vi "read file.vi"() -> ()   [LabVIEW 2011]
panel:
  out "Image":T1(plugin-control)
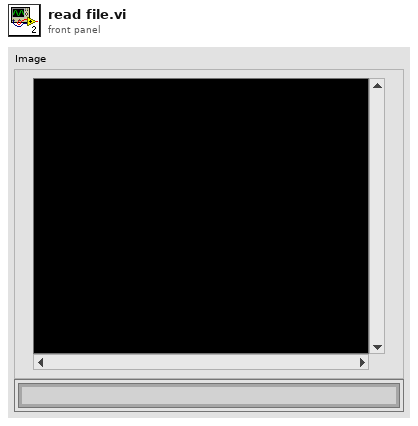
[diagram p1: front panel]
types:
  T1 = typedef "IMAQ Image.ctl" = refnum<image>
  T2 = typedef "Image Type" = u32
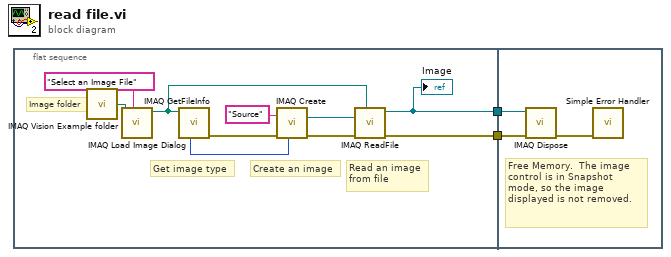
[diagram p0: block diagram]
diagram:
  n1 = flat-sequence {
    tunnel: [w5] -> w2
    tunnel: [w4] -> w1
    tunnel: w2 -> [w15]
    tunnel: w1 -> [w13]
    frame #0 {
      # "Get image type"
      # "Image folder"
      # "Read an image\nfrom file"
      # "Create an image"
      n2 = call "IMAQ Vision Example folder.vi"() -> ("Example Image Path"=w9:path)  [unwired: 1 out]
      n3 = call "IMAQ Load Image Dialog"("Prompt"="Select an Image File" ("prompt"), "Start Path"=w9) -> ("Path"=w3:path)  [unwired: 5 in, 4 out]
      n4 = call "IMAQ GetFileInfo"("File Path"=w3) -> ("error out"=w7:errorcluster, "Image Type"=w8:T2)  [unwired: 1 in, 8 out]
      n5 = call "IMAQ Create"("Image Name"="Source", "Image Type"=w8, "error in (no error)"=w7) -> ("New Image"=w11:T1, "error out"=w12:errorcluster)  [unwired: 1 in, 1 out]
      n6 = call "IMAQ ReadFile"("File Path"=w3, "error in (no error)"=w12, "Image"=w11) -> ("error out"=w5:errorcluster, "Image Out"=w4:T1)  [unwired: 2 in, 5 out]
      "Image" <- w4
    }
    frame #1 {
      # "Free Memory.  The image control is in Snapshot mode, so the image displayed is not removed."
      n7 = call "IMAQ Dispose"("Image"=w13, "error in (no error)"=w15) -> ("error out"=w14:errorcluster)  [unwired: 1 in, 3 out]
      n8 = call <vilib>:"Simple Error Handler.vi"("error in (no error)"=w14) -> ()  [unwired: 1 in, 8 out]
    }
  }
